vi "CHD_DRIVE_GET_MAX.vi"() -> (3 "Max Wheel Vel (Meter/Sec)":dbl)   [LabVIEW 2019]
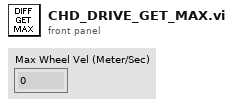
[diagram p1: front panel]
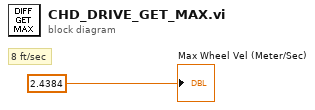
[diagram p0: block diagram]
diagram:
  # "8 ft/sec"
  "Max Wheel Vel (Meter/Sec)" <- 2.4384
